vi "Configure Clock.vi"(0 "VISA resource name":refnum<visa-resource-name>, 1 "Set Current Time (Yes)":bool=TRUE, 5 "Hour (12)":i32=12 min=0 max=23 step=1, 7 "Minutes (12)":i32=12 min=0 max=59 step=1 format="%02.0f", 9 "Time Format (AM)":u16(ring) items=["AM", "PM", "24 Hr Format"], 11 "error in (no error)":errorcluster) -> (4 "VISA resource name out":refnum<visa-resource-name>, 15 "error out":errorcluster)   [LabVIEW 2016, in "EFD Ultimus V.lvlib"]
doc: "Sets the time on the real time clock on the Ultimus V.\nIf set to Current Time is set to TRUE, then the current system Time will be used.\nHost Format: EB--HhhMmmAMa\n hh:Hours. 0-23 for 24 hour format, 1-12 for 12 Hour Format\n mm:minutes. 0-59\n a: Hour Format. 0=AM, 1=PM, 2=24 Hr Format"
uses:
  EFD Ultimus V.lvlib
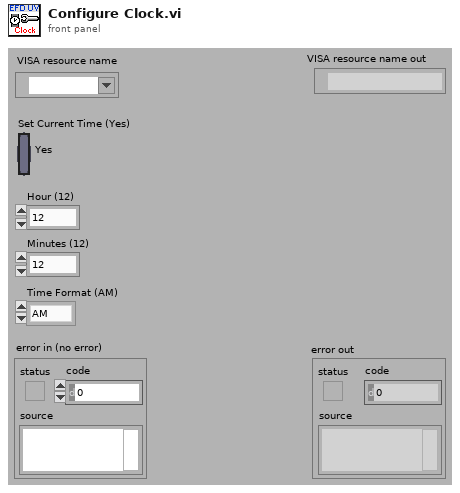
[diagram p1: front panel]
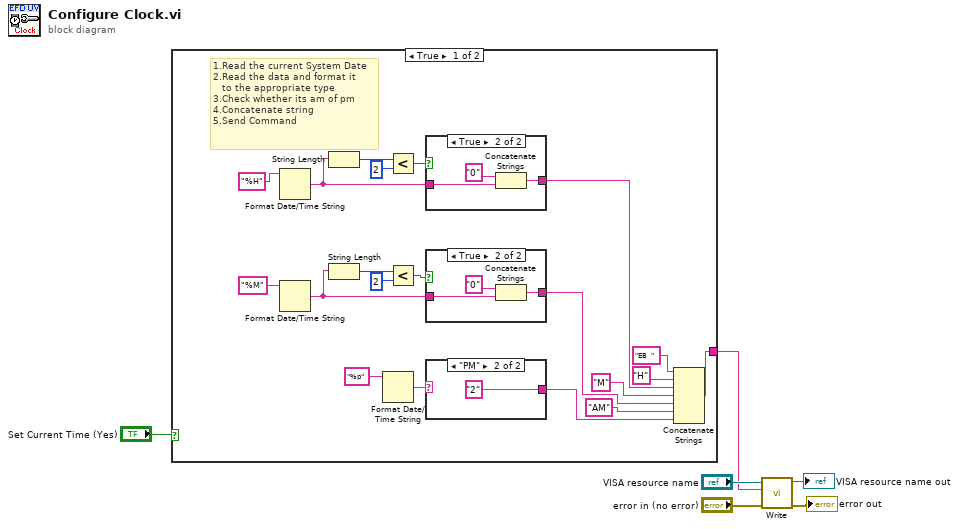
[diagram p0: block diagram]
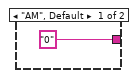
[diagram p4: hidden frame]
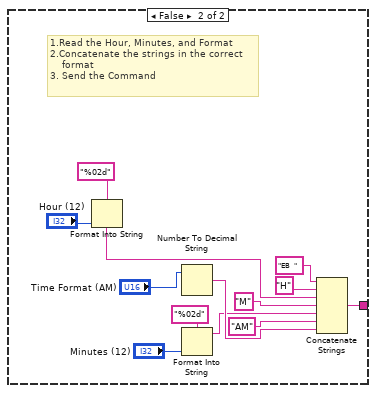
[diagram p5: hidden frame]
diagram:
  n1 = case shown="True" "Set Current Time (Yes)" {
    tunnel: [w22 w47] -> w3
    frame True {
      # "1.Read the current System Date\n2.Read the data and format it\n   to the appropriate type\n3.Check whether its am of pm\n4.Concatenate string\n5.Send Command"
      n2 = Format Date/Time String(time format string (%c)="%H") -> (date/time string=w13:string)  [unwired: 2 out]
      n3 = Format Date/Time String(time format string (%c)="%M") -> (date/time string=w8:string)  [unwired: 2 out]
      n4 = String Length(string=w13) -> (length=w16:i32)
      n5 = String Length(string=w8) -> (length=w10:i32)
      n6 = Format Date/Time String(time format string (%c)="%p") -> (date/time string=w17:string)  [unwired: 2 out]
      n7 = Less?(x=w16, y=2) -> (x < y?=w14:bool)
      n8 = Less?(x=w10, y=2) -> (x < y?=w9:bool)
      n9 = case shown="True" w14 {
        tunnel: w13 -> [w31 w34]
        tunnel: [w31 w32] -> w12
        frame False {
        }
        frame True {
          n10 = Concatenate Strings("0" ("string"), w34) -> (w32:string)
        }
      }
      n11 = case shown="True" w9 {
        tunnel: [w27 w29] -> w7
        tunnel: w8 -> [w27 w28]
        frame False {
        }
        frame True {
          n12 = Concatenate Strings("0" ("string"), w28) -> (w29:string)
        }
      }
      n13 = case shown="\"PM\"" w17 {
        tunnel: ["0" ("string") "2" ("string")] -> w21
        frame "AM", Default {
        }
        frame "PM" {
        }
      }
      n14 = Concatenate Strings("EB  " ("string"), "H" ("string"), w12, "M" ("string"), w7, "AM" ("string"), w21) -> (w22:string)
    }
    frame False {
      # "1.Read the Hour, Minutes, and Format\n2.Concatenate the strings in the correct\n    format\n3. Send the Command"
      n15 = Format Into String(format string="%02d", "Hour (12)") -> (resulting string=w37:string)  [unwired: 2 in, 1 out]
      n16 = Number To Decimal String(number="Time Format (AM)") -> (decimal integer string=w43:string)  [unwired: 1 in]
      n17 = Format Into String(format string="%02d", "Minutes (12)") -> (resulting string=w40:string)  [unwired: 2 in, 1 out]
      n18 = Concatenate Strings("EB  " ("string"), "H" ("string"), w37, "M" ("string"), w40, "AM" ("string"), w43) -> (w47:string)
    }
  }
  n19 = call "Write.vi"("error in (no error)"="error in (no error)", "Command To Write"=w3, "VISA resource name"="VISA resource name") -> ("error out"=→"error out":errorcluster, "VISA resource name out"=→"VISA resource name out":refnum<visa-resource-name>)  [unwired: 7 out]
